vi "alpha_0.3.vi"() -> ()   [LabVIEW 2018]
panel:
  in  "Rácio de entrada":dbl
  out "Tempo no Verde + Amarelo":dbl caption="Elapsed Time (s)"
  out "Tempo no Vermelho":dbl caption="Elapsed Time (s)"
  out "Congestionamento  2":bool
  out "Congestionamento 1":bool
  in  "Slide 2":dbl(slide) scale=0.0..10.0
  in  "Slide 1":dbl(slide) scale=0.0..10.0
  in  "Caso de emergência":bool
  out "GreenP 2":bool
  out "RedP 2":bool
  out "GreenP 1":bool
  out "RedP 1":bool
  in  "Estado 2":dbl
  out "Velocidade excedida 3":bool
  in  "Velocidade 3":dbl
  out "RED 4":bool
  out "YELLOW 4":bool
  out "GREEN 4":bool
  out "Velocidade excedida 2":bool
  in  "Velocidade 2":dbl
  out "RED 3":bool
  out "YELLOW 3":bool
  out "GREEN 3":bool
  in  "stop":bool
  in  "Timer (s)":dbl
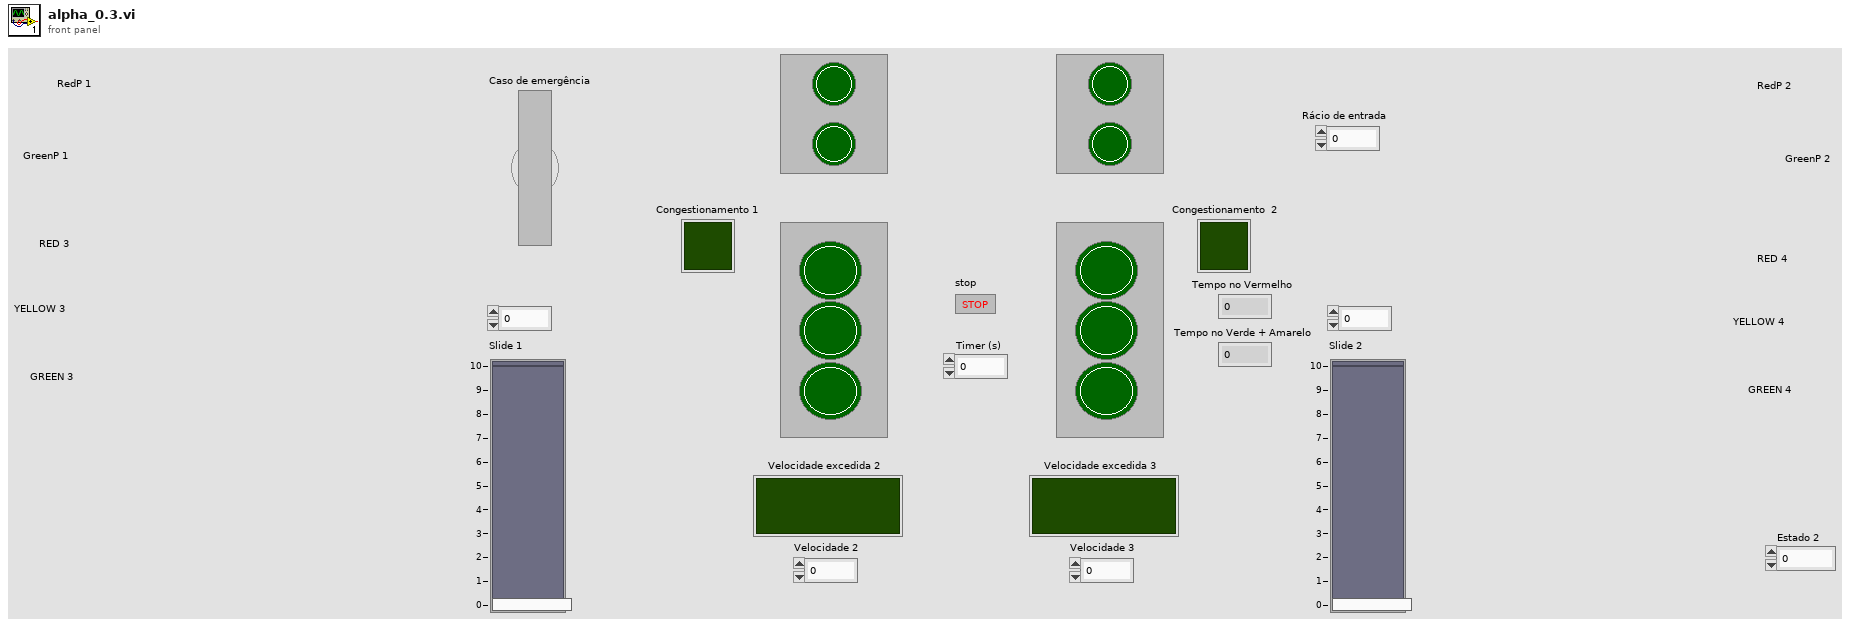
[diagram p1: front panel]
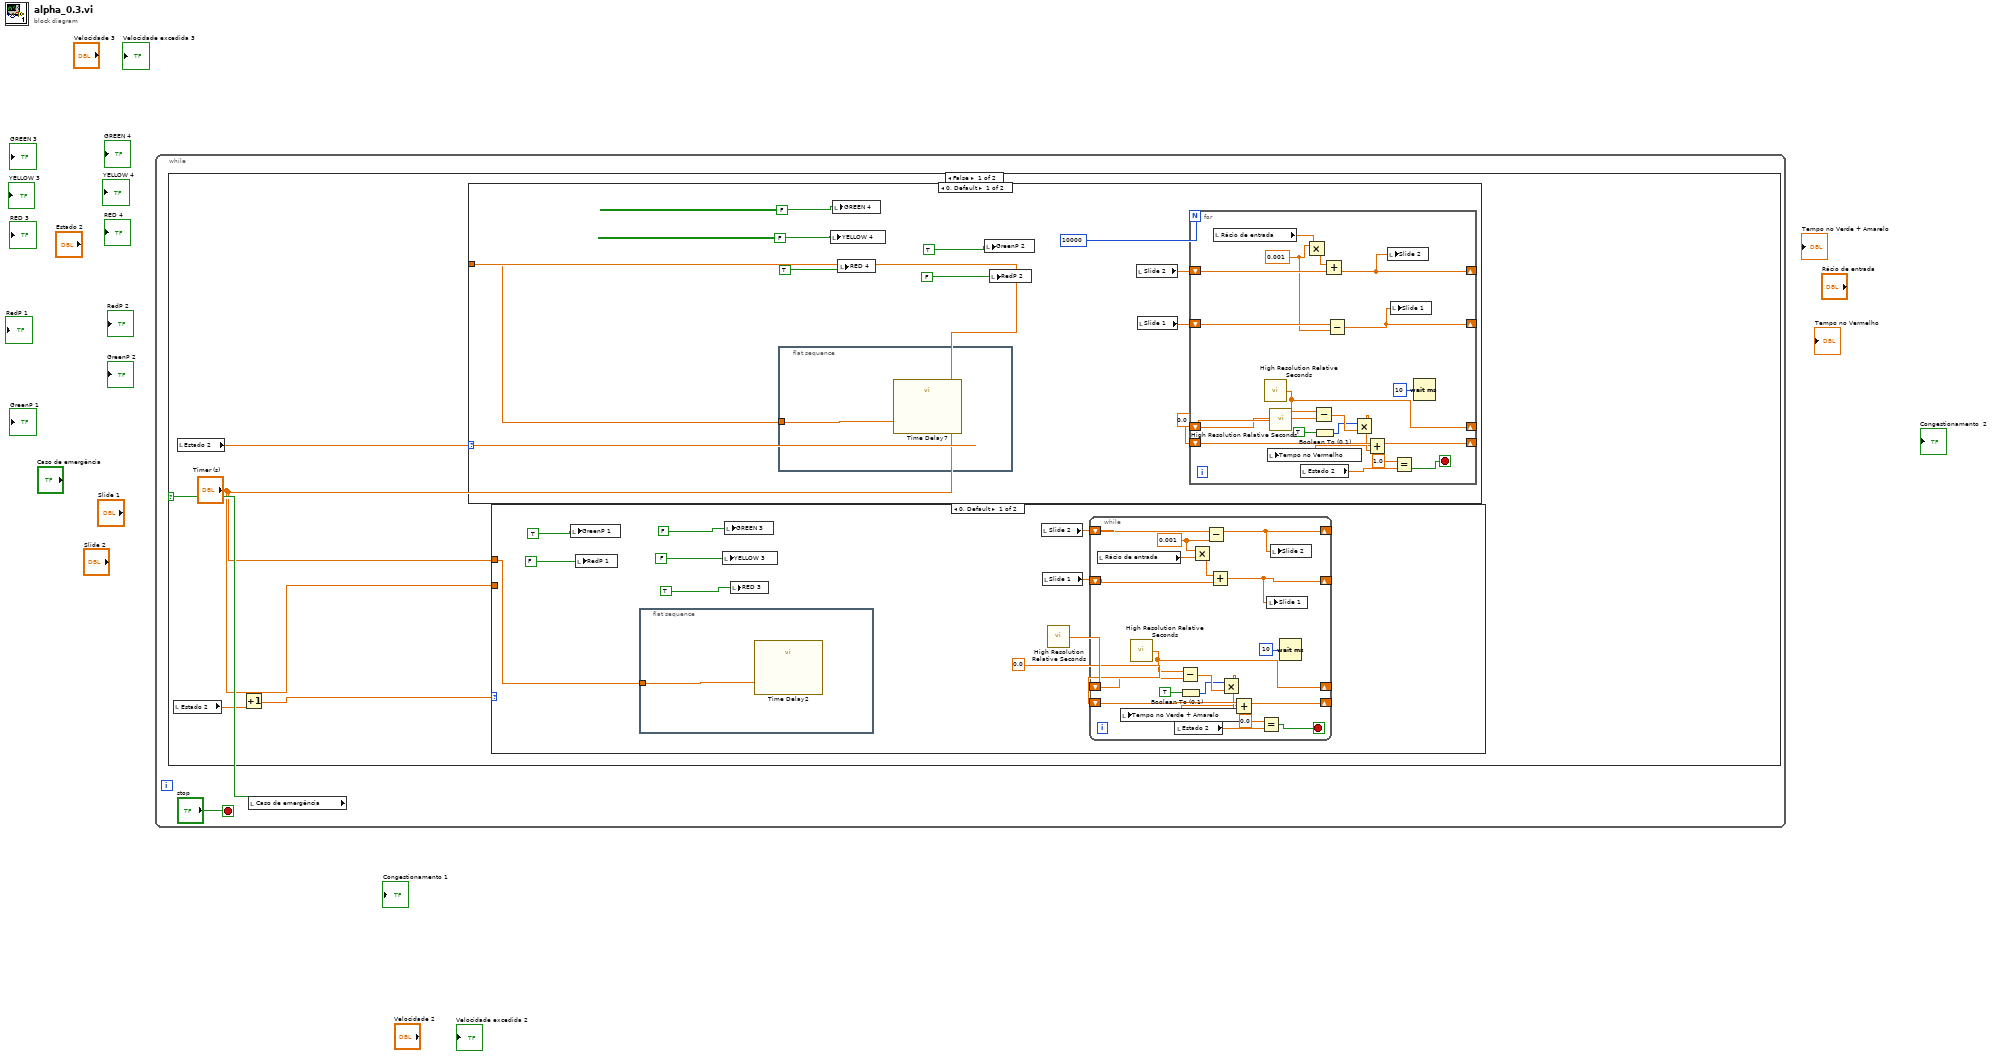
[diagram p0: block diagram]
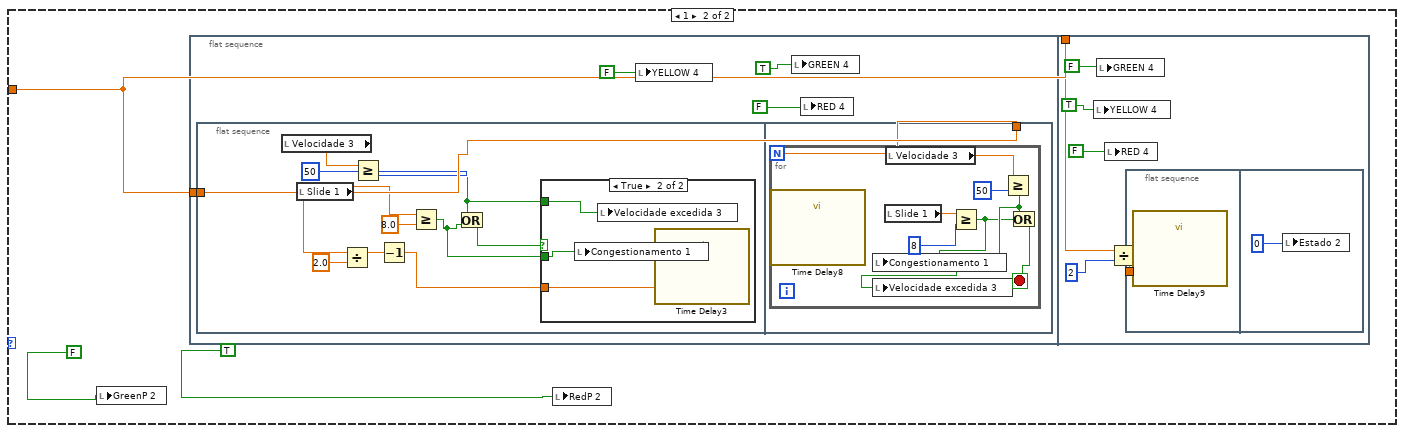
[diagram p2: hidden frame]
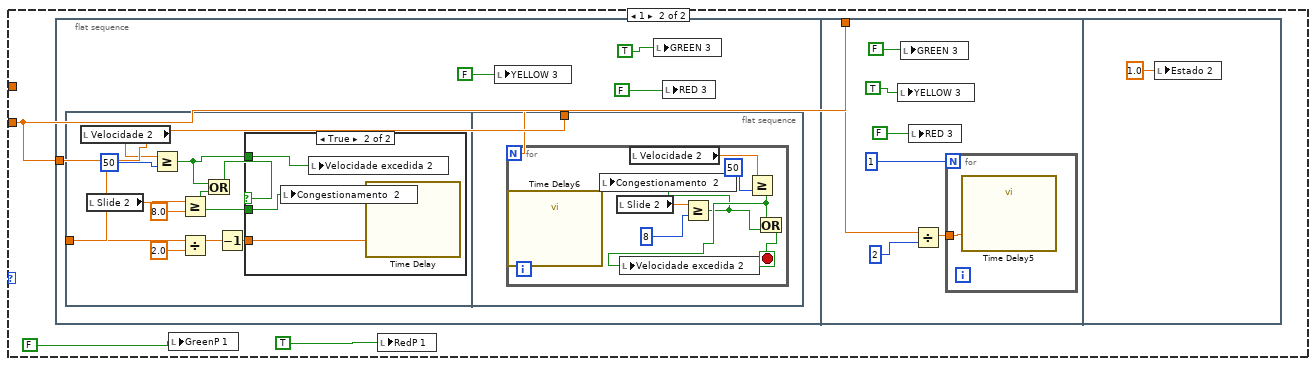
[diagram p4: hidden frame]
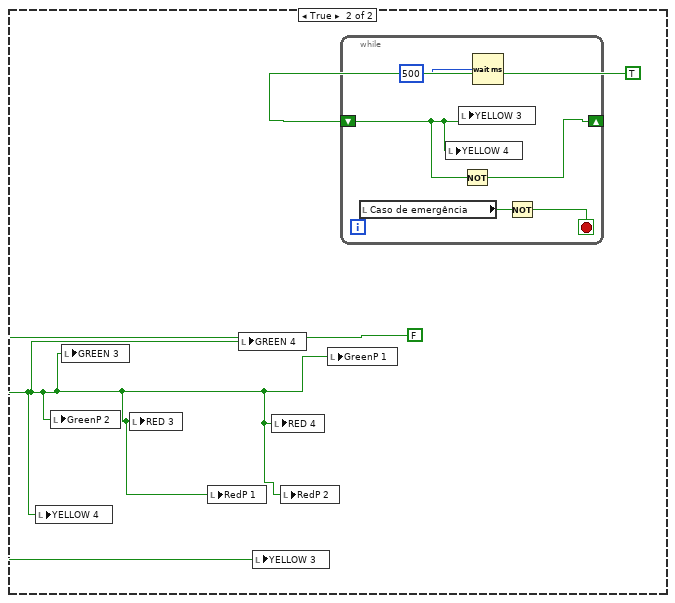
[diagram p6: hidden frame]
diagram:
  n1 = while {
    stop <- "stop" stop-if-true
    n2 = local read "Caso de emergência"() -> (w1:bool)
    n3 = case shown="False" w1 {
      frame False {
        n4 = local read "Estado 2"() -> (w6:dbl)
        n5 = local read "Estado 2"() -> (w4:dbl)
        n6 = Increment(x=w6) -> (x+1=w5:dbl)
        n7 = case shown="0, Default" w4 {
          tunnel: "Timer (s)" -> [w12 w40]
          frame 0, Default {
            n8 = flat-sequence {
              tunnel: w12 -> [w37]
              frame #0 {
                n9 = call "Time Delay7"("Delay Time (s)"=w37) -> ()  [unwired: 10 in, 1 out]
              }
            }
            n10 = local write "YELLOW 4"(FALSE) -> ()
            n11 = local write "GREEN 4"(FALSE) -> ()
            n12 = local write "RED 4"(TRUE) -> ()
            n13 = local write "GreenP 2"(TRUE) -> ()
            n14 = local write "RedP 2"(FALSE) -> ()
            n15 = local read "Slide 2"() -> (w7:dbl)
            n16 = local read "Slide 1"() -> (w8:dbl)
            n17 = call <vilib>:"High Resolution Relative Seconds.vi"() -> ("relative seconds"=w11:dbl)
            n18 = for {
              N: 10000 -> [_]
              shift-right: [w34] -> _
              shift-left: w11 -> [w35]
              shift-right: [w28] -> _
              shift-left: 0.0 -> [w33]
              shift-right: [w22] -> _
              shift-left: w7 -> [w24]
              shift-right: [w20] -> _
              shift-left: w8 -> [w19]
              stop <- w26 stop-if-true
              w18 = 0.001 ("x")
              n19 = local read "Rácio de entrada"() -> (w23:dbl)
              n20 = call <vilib>:"High Resolution Relative Seconds.vi"() -> ("relative seconds"=w34:dbl)
              n21 = local read "Estado 2"() -> (w27:dbl)
              n22 = Multiply(x=w18, y=w23) -> (x*y=w21:dbl)
              n23 = Subtract(x=w34, y=w35) -> (x-y=w31:dbl)
              n24 = Boolean To (0,1)(Boolean=TRUE) -> (0, 1=w29:i16)
              n25 = Add(x=w21, y=w24) -> (x+y=w22:dbl)
              n26 = Subtract(x=w19, y=w18) -> (x-y=w20:dbl)
              n27 = Multiply(x=w29, y=w31) -> (x*y=w30:dbl)
              n28 = Add(x=w33, y=w30) -> (x+y=w28:dbl)
              n29 = local write "Tempo no Vermelho"(w28) -> ()
              n30 = local write "Slide 2"(w22) -> ()
              n31 = local write "Slide 1"(w20) -> ()
              n32 = Equal?(x=1.0, y=w27) -> (x = y?=w26:bool)
              n33 = Wait (ms)(milliseconds to wait=u32 10) -> ()  [unwired: 1 out]
            }
          }
          frame 1 {
            n34 = local write "GreenP 2"(FALSE) -> ()
            n35 = flat-sequence {
              tunnel: w40 -> [w41]
              tunnel: w40 -> [w68]
              frame #0 {
                n36 = flat-sequence {
                  tunnel: w41 -> [w50]
                  tunnel: w41 -> [w59]
                  frame #0 {
                    n37 = local read "Velocidade 3"() -> (w53:dbl)
                    n38 = local read "Slide 1"() -> (w47:dbl)
                    n39 = Divide(x=w50, y=2.0) -> (x/y=w54:dbl)
                    n40 = Greater Or Equal?(x=w53, y=50) -> (x >= y?=w46:bool)
                    n41 = Decrement(x=w54) -> (x-1=w55:dbl)
                    n42 = Greater Or Equal?(x=w47, y=8.0) -> (x >= y?=w45:bool)
                    n43 = Or(x=w46, y=w45) -> (x .or. y?=w48:bool)
                    n44 = case shown="True" w48 {
                      tunnel: w55 -> [_ w58]
                      tunnel: w46 -> [_ w57]
                      tunnel: w45 -> [_ w56]
                      frame False {
                      }
                      frame True {
                        n45 = local write "Congestionamento 1"(w56) -> ()
                        n46 = local write "Velocidade excedida 3"(w57) -> ()
                        n47 = call "Time Delay3"("Delay Time (s)"=w58) -> ()  [unwired: 10 in, 1 out]
                      }
                    }
                  }
                  frame #1 {
                    n48 = for {
                      N: w59 -> [_]
                      stop <- w64 stop-if-true
                      n49 = call "Time Delay8"() -> ()  [unwired: 11 in, 1 out]
                      n50 = local read "Slide 1"() -> (w63:dbl)
                      n51 = local read "Velocidade 3"() -> (w66:dbl)
                      n52 = Greater Or Equal?(x=w63, y=8) -> (x >= y?=w60:bool)
                      n53 = local write "Congestionamento 1"(w60) -> ()
                      n54 = Greater Or Equal?(x=w66, y=50) -> (x >= y?=w61:bool)
                      n55 = local write "Velocidade excedida 3"(w61) -> ()
                      n56 = Or(x=w61, y=w60) -> (x .or. y?=w64:bool)
                    }
                  }
                }
                n57 = local write "YELLOW 4"(FALSE) -> ()
                n58 = local write "GREEN 4"(TRUE) -> ()
                n59 = local write "RED 4"(FALSE) -> ()
              }
              frame #1 {
                n60 = local write "YELLOW 4"(TRUE) -> ()
                n61 = local write "GREEN 4"(FALSE) -> ()
                n62 = local write "RED 4"(FALSE) -> ()
                n63 = Divide(x=w68, y=2) -> (x/y=w67:dbl)
                n64 = flat-sequence {
                  tunnel: w67 -> [w73]
                  frame #0 {
                    n65 = call "Time Delay9"("Delay Time (s)"=w73) -> ()  [unwired: 10 in, 1 out]
                  }
                  frame #1 {
                    n66 = local write "Estado 2"(0) -> ()
                  }
                }
              }
            }
            n67 = local write "RedP 2"(TRUE) -> ()
          }
        }
        n68 = case shown="0, Default" w5 {
          tunnel: "Timer (s)" -> [_ w105]
          tunnel: "Timer (s)" -> [w76 _]
          frame 0, Default {
            n69 = local write "GreenP 1"(TRUE) -> ()
            n70 = local write "RedP 1"(FALSE) -> ()
            n71 = flat-sequence {
              tunnel: w76 -> [w85]
              frame #0 {
                n72 = call "Time Delay2"("Delay Time (s)"=w85) -> ()  [unwired: 10 in, 1 out]
              }
            }
            n73 = local write "YELLOW 3"(FALSE) -> ()
            n74 = local write "GREEN 3"(FALSE) -> ()
            n75 = local write "RED 3"(TRUE) -> ()
            n76 = local read "Slide 2"() -> (w77:dbl)
            n77 = local read "Slide 1"() -> (w75:dbl)
            n78 = call <vilib>:"High Resolution Relative Seconds.vi"() -> ("relative seconds"=w79:dbl)
            n79 = while {
              shift-right: [w102] -> _
              shift-left: w79 -> [w103]
              shift-right: [w96] -> _
              shift-left: 0.0 -> [w101]
              shift-right: [w91] -> _
              shift-left: w77 -> [w92]
              shift-right: [w86] -> _
              shift-left: w75 -> [w87]
              stop <- w94 stop-if-true
              w90 = 0.001 ("y")
              n80 = local read "Rácio de entrada"() -> (w89:dbl)
              n81 = call <vilib>:"High Resolution Relative Seconds.vi"() -> ("relative seconds"=w102:dbl)
              n82 = local read "Estado 2"() -> (w95:dbl)
              n83 = Subtract(x=w102, y=w103) -> (x-y=w99:dbl)
              n84 = Boolean To (0,1)(Boolean=TRUE) -> (0, 1=w97:i16)
              n85 = Multiply(x=w90, y=w89) -> (x*y=w88:dbl)
              n86 = Subtract(x=w92, y=w90) -> (x-y=w91:dbl)
              n87 = Add(x=w88, y=w87) -> (x+y=w86:dbl)
              n88 = Multiply(x=w97, y=w99) -> (x*y=w98:dbl)
              n89 = Add(x=w101, y=w98) -> (x+y=w96:dbl)
              n90 = local write "Tempo no Verde + Amarelo"(w96) -> ()
              n91 = Equal?(x=0.0, y=w95) -> (x = y?=w94:bool)
              n92 = local write "Slide 1"(w86) -> ()
              n93 = local write "Slide 2"(w91) -> ()
              n94 = Wait (ms)(milliseconds to wait=u32 10) -> ()  [unwired: 1 out]
            }
          }
          frame 1 {
            n95 = flat-sequence {
              tunnel: w105 -> [w108]
              tunnel: w105 -> [w134]
              frame #0 {
                n96 = flat-sequence {
                  tunnel: w108 -> [w120]
                  tunnel: w108 -> [w126]
                  frame #0 {
                    n97 = local read "Velocidade 2"() -> (w122:dbl)
                    n98 = local read "Slide 2"() -> (w115:dbl)
                    n99 = Greater Or Equal?(x=w122, y=50) -> (x >= y?=w113:bool)
                    n100 = Greater Or Equal?(x=w115, y=8.0) -> (x >= y?=w112:bool)
                    n101 = Divide(x=w120, y=2.0) -> (x/y=w119:dbl)
                    n102 = Or(x=w113, y=w112) -> (x .or. y?=w116:bool)
                    n103 = Decrement(x=w119) -> (x-1=w117:dbl)
                    n104 = case shown="True" w116 {
                      tunnel: w117 -> [_ w125]
                      tunnel: w113 -> [_ w124]
                      tunnel: w112 -> [_ w123]
                      frame False {
                      }
                      frame True {
                        n105 = local write "Congestionamento  2"(w123) -> ()
                        n106 = local write "Velocidade excedida 2"(w124) -> ()
                        n107 = call "Time Delay"("Delay Time (s)"=w125) -> ()  [unwired: 10 in, 1 out]
                      }
                    }
                  }
                  frame #1 {
                    n108 = for {
                      N: w126 -> [_]
                      stop <- w129 stop-if-true
                      n109 = call "Time Delay6"() -> ()  [unwired: 11 in, 1 out]
                      n110 = local read "Slide 2"() -> (w131:dbl)
                      n111 = local read "Velocidade 2"() -> (w133:dbl)
                      n112 = Greater Or Equal?(x=w131, y=8) -> (x >= y?=w127:bool)
                      n113 = local write "Congestionamento  2"(w127) -> ()
                      n114 = Greater Or Equal?(x=w133, y=50) -> (x >= y?=w128:bool)
                      n115 = local write "Velocidade excedida 2"(w128) -> ()
                      n116 = Or(x=w128, y=w127) -> (x .or. y?=w129:bool)
                    }
                  }
                }
                n117 = local write "YELLOW 3"(FALSE) -> ()
                n118 = local write "GREEN 3"(TRUE) -> ()
                n119 = local write "RED 3"(FALSE) -> ()
              }
              frame #1 {
                n120 = local write "YELLOW 3"(TRUE) -> ()
                n121 = local write "GREEN 3"(FALSE) -> ()
                n122 = local write "RED 3"(FALSE) -> ()
                n123 = Divide(x=w134, y=2) -> (x/y=w137:dbl)
                n124 = for {
                  N: 1 -> [_]
                  tunnel: w137 -> [w141]
                  n125 = call "Time Delay5"("Delay Time (s)"=w141) -> ()  [unwired: 10 in, 1 out]
                }
              }
              frame #2 {
                n126 = local write "Estado 2"(1.0 ("Estado 2")) -> ()
              }
            }
            n127 = local write "GreenP 1"(FALSE) -> ()
            n128 = local write "RedP 1"(TRUE) -> ()
          }
        }
      }
      frame True {
        w143 = FALSE
        n129 = local write "YELLOW 4"(w143) -> ()
        n130 = local write "GreenP 2"(w143) -> ()
        n131 = local write "GREEN 3"(w143) -> ()
        n132 = local write "RED 3"(w143) -> ()
        n133 = local write "RedP 1"(w143) -> ()
        n134 = local write "GREEN 4"(w143) -> ()
        n135 = local write "YELLOW 3"(w143) -> ()
        n136 = local write "RED 4"(w143) -> ()
        n137 = local write "RedP 2"(w143) -> ()
        n138 = local write "GreenP 1"(w143) -> ()
        n139 = while {
          shift-right: [w149] -> _
          shift-left: TRUE -> [w145]
          stop <- w146 stop-if-true
          n140 = local read "Caso de emergência"() -> (w147:bool)
          n141 = local write "YELLOW 4"(w145) -> ()
          n142 = local write "YELLOW 3"(w145) -> ()
          n143 = Not(x=w145) -> (.not. x?=w149:bool)
          n144 = Wait (ms)(milliseconds to wait=500) -> ()  [unwired: 1 out]
          n145 = Not(x=w147) -> (.not. x?=w146:bool)
        }
      }
    }
  }
